vi "Convex Hull.vi"(10 "Y":dbl[](array[numeric]), 11 "X":dbl[](array[numeric])) -> (0 "error":i32, 3 "Convex Hull":i32[](array[numeric]))   [LabVIEW 2020, in "NI_AAL_Geometry.lvlib"]
doc: "Computes the vertices of a convex polygon, which are the set of points that make up the polygon that contains all the points."
uses:
  <vilib>/Analysis/NI_AAL_Geometry.lvlib
panel:
  # "Convex Hull"
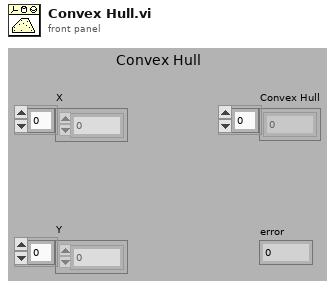
[diagram p1: front panel]
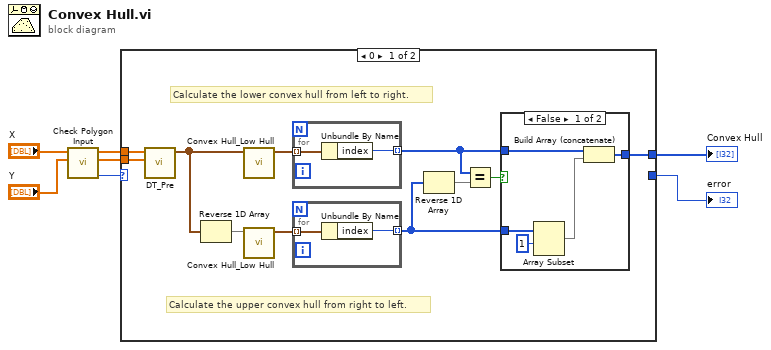
[diagram p0: block diagram]
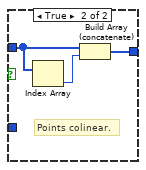
[diagram p2: hidden frame]
diagram:
  n1 = call <vilib>:"Check Polygon Input.vi"("Y In"="Y", "X In"="X") -> ("error"=w1:i32, "Y Out"=w4:dbl[], "X Out"=w5:dbl[])  [unwired: 7 in]
  n2 = case shown="0" w1 {
    selector: w1 -> [_ w31]
    tunnel: w5 -> [w18 _]
    tunnel: w4 -> [w17 _]
    tunnel: [_ w31] -> w2
    tunnel: [w10 _] -> w3
    frame 0 {
      # "Calculate the upper convex hull from right to left."
      # "Calculate the lower convex hull from left to right."
      n3 = call <vilib>:"DT_Pre.vi"("Y"=w17, "X"=w18) -> ("Points"=w15:cluster{"x":dbl, "y":dbl, "index":i32}[])  [unwired: 7 in, 2 out]
      n4 = Reverse 1D Array(array=w15) -> (reversed array=w16:cluster{"x":dbl, "y":dbl, "index":i32}[])
      n5 = call <vilib>:"Convex Hull_Low Hull.vi"("Points"=w15) -> ("Low Hull"=w14:cluster{"x":dbl, "y":dbl, "index":i32}[])  [unwired: 10 in]
      n6 = call <vilib>:"Convex Hull_Low Hull.vi"("Points"=w16) -> ("Low Hull"=w9:cluster{"x":dbl, "y":dbl, "index":i32}[])  [unwired: 10 in]
      n7 = for {
        tunnel: w14 -> [w30] mode=indexing
        tunnel: [w29] -> w12 mode=indexing
        n8 = Unbundle By Name(w30) -> ("index"=w29:i32)
      }
      n9 = for {
        tunnel: w9 -> [w20] mode=indexing
        tunnel: [w19] -> w8 mode=indexing
        n10 = Unbundle By Name(w20) -> ("index"=w19:i32)
      }
      n11 = Reverse 1D Array(array=w8) -> (reversed array=w11:i32[])
      n12 = Equal?(x=w12, y=w11) -> (x = y?=w13:bool)
      n13 = case shown="False" w13 {
        tunnel: w12 -> [w25 w28]
        tunnel: w8 -> [w24 _]
        tunnel: [w21 w26] -> w10
        frame False {
          n14 = Array Subset(array=w24, index=1) -> (w22:i32[])  [unwired: 1 in]
          n15 = Build Array (concatenate)(w25, w22) -> (w21:i32[])
        }
        frame True {
          # "Points colinear."
          n16 = Index Array(array=w28) -> (element=w27:i32)  [unwired: 1 in]
          n17 = Build Array (concatenate)(w28, w27) -> (w26:i32[])
        }
      }
    }
    frame -1, Default {
    }
  }
  "Convex Hull" <- w3
  "error" <- w2
